vi "Zero Fetch.vi"(8 "error in (no error)":errorcluster, 10 "firmware revision":string(combo), 11 "VISA resource name":refnum<visa-resource-name>) -> (0 "error out":errorcluster, 2 "bridge error":T1, 3 "VISA resource name out":refnum<visa-resource-name>)   [LabVIEW 2021, in "Andeen-Hagerling 2700A.lvlib"]
doc: "Provides an automatic way to enter capacitance and loss Zero\ncompensation values."
uses:
  Andeen-Hagerling 2700A.lvlib
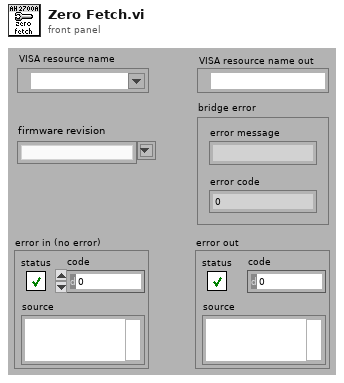
[diagram p1: front panel]
types:
  T1 = cluster{"error message":string, "error code":i32}
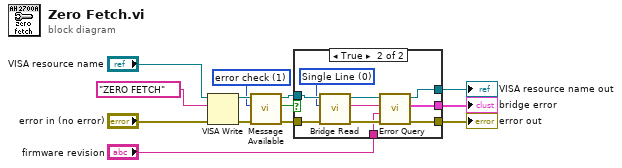
[diagram p0: block diagram]
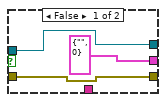
[diagram p2: hidden frame]
diagram:
  w1 = u16 1 items=["none", "error check", "multiline read", "infinite"] ("delay")
  n1 = VISA Write(VISA resource name="VISA resource name", write buffer="ZERO FETCH" ("command"), error in (no error)="error in (no error)") -> (VISA resource name out=w7:refnum<visa-resource-name>, error out=w6:errorcluster)  [unwired: 1 out]
  n2 = call "Message Available.vi"("error in (no error)"=w6, "delay"=w1, "VISA resource name"=w7) -> ("error out"=w8:errorcluster, "message available"=w10:bool, "VISA resource name out"=w9:refnum<visa-resource-name>)  [unwired: 6 in]
  n3 = case shown="True" w10 {
    tunnel: w9 -> [w15 w23]
    tunnel: w8 -> [w16 w22]
    tunnel: "firmware revision" -> [_ w21]
    tunnel: [w16 w20] -> w4
    tunnel: [w15 w19] -> w3
    tunnel: [T1 {"error message"="", "error code"=0} ("bridge error") w18] -> w2
    frame False {
    }
    frame True {
      w17 = u16 0 items=["Single Line", "Multi-Line"] ("Multiline")
      n4 = call "Bridge Read.vi"("error in (no error)"=w22, "multiline"=w17, "VISA resource name"=w23) -> ("error out"=w25:errorcluster, "read buffer"=w26:string, "VISA resource name out"=w24:refnum<visa-resource-name>)  [unwired: 6 in]
      n5 = call "Error Query.vi"("error in (no error)"=w25, "firmware revision"=w21, "measurement line"=w26, "VISA resource name"=w24) -> ("error out"=w20:errorcluster, "bridge error"=w18:T1, "VISA resource name out"=w19:refnum<visa-resource-name>)  [unwired: 5 in]
    }
  }
  "VISA resource name out" <- w3
  "error out" <- w4
  "bridge error" <- w2
